vi "Load Measurement Definitions.vi"(8 "error in (no error)":errorcluster, 11 "NI Generic Parser in":refnum<class "NI Generic Parser.lvclass">=refnum) -> (0 "error out":errorcluster, 3 "NI Generic Parser out":refnum<class "NI Generic Parser.lvclass">)   [LabVIEW 2018, in "NI Generic Parser.lvlib" / "NI Generic Parser.lvclass"]
uses:
  NI Generic Parser.lvclass
  <vilib>/ErrorRing/Error Ring.xnode
  <vilib>/Utility/error.llb/Error Cluster From Error Code.vi
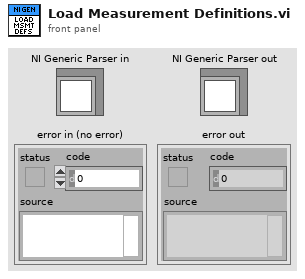
[diagram p1: front panel]
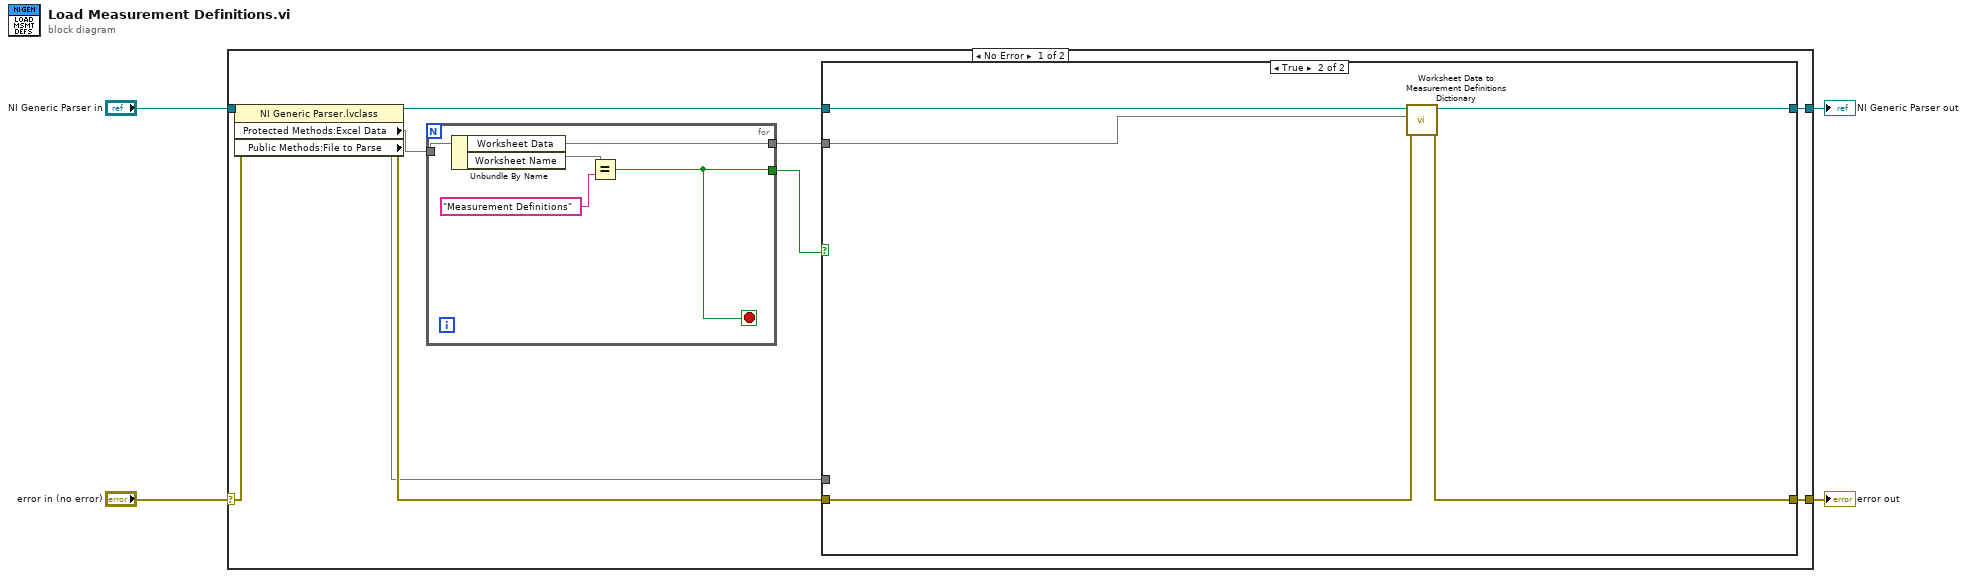
[diagram p0: block diagram]
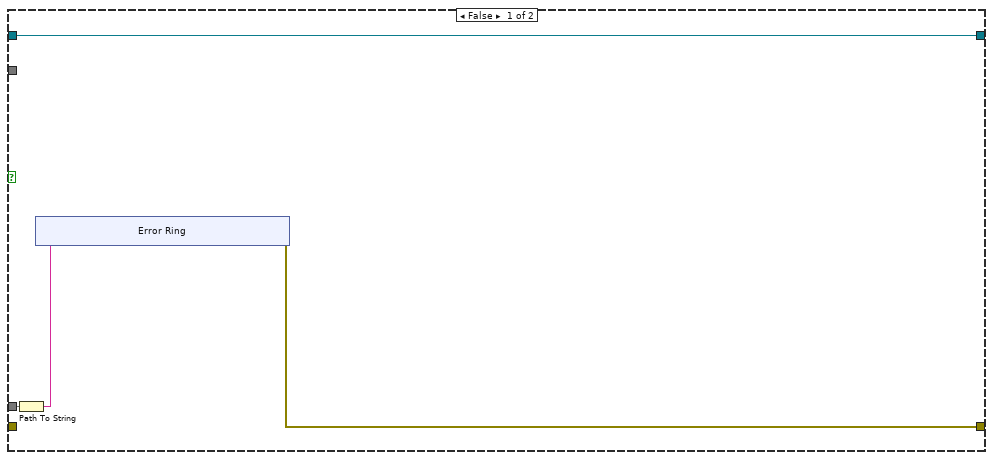
[diagram p2: hidden frame]
diagram:
  n1 = case shown="No Error" "error in (no error)" {
    selector: "error in (no error)" -> [w14 w37]
    tunnel: [w8 w37] -> w3
    tunnel: [w5 w36] -> w1
    tunnel: "NI Generic Parser in" -> [w13 w36]
    frame No Error {
      n2 = property class="NI Generic Parser.lvclass"(reference=w13, error in=w14) -> (reference out=w6:refnum<class "NI Generic Parser.lvclass">, error out=w11:errorcluster, "Protected Methods:Excel Data"=w12, "Public Methods:File to Parse"=w9)
      n3 = for {
        tunnel: w12 -> [w35]
        tunnel: [w32] -> w7
        tunnel: [w31] -> w10
        stop <- w31 stop-if-true
        n4 = Unbundle By Name(w35) -> ("Worksheet Data"=w32, "Worksheet Name"=w34)
        n5 = Equal?(x=w34, y="Measurement Definitions") -> (x = y?=w31:bool)
      }
      n6 = case shown="True" w10 {
        tunnel: w11 -> [_ w27]
        tunnel: w9 -> [w18 _]
        tunnel: [w16 w26] -> w8
        tunnel: w7 -> [_ w30]
        tunnel: w6 -> [w15 w29]
        tunnel: [w15 w28] -> w5
        frame False {
          n7 = Path To String(path=w18) -> (string=w17:string)
          n8 = xnode "Error Ring"("parameter 0"=w17) -> ("error out"=w16:errorcluster)
        }
        frame True {
          n9 = call "Worksheet Data to Measurement Definitions Dictionary.vi"("error in (no error)"=w27, "Worksheet Data"=w30, "NI Generic Parser in"=w29) -> ("error out"=w26:errorcluster, "NI Generic Parser out"=w28:refnum<class "NI Generic Parser.lvclass">)  [unwired: 7 in]
        }
      }
    }
    frame Error {
    }
  }
  "error out" <- w3
  "NI Generic Parser out" <- w1
